vi "Code 0.0.2.vi"() -> ()   [LabVIEW 2017]
uses:
  <vilib>/Instr/_visa.llb/VISA Configure Serial Port (Instr).vi
panel:
  out "Error List":string
  in  "Flash Baudrate":u32(ring)=115200 items=["4800"=4800, "9600"=9600, "19200"=19200, "38400"=38400, "57600"=57600, "115200"=115200, "230400"=230400, "460800"=460800, "921600"=921600]
  in  "cmd Baudrate":u32(ring)=230400 items=["4800"=4800, "9600"=9600, "19200"=19200, "38400"=38400, "57600"=57600, "115200"=115200, "230400"=230400, "460800"=460800, "921600"=921600]
  in  "UUT COM Port":refnum<visa-resource-name>="COM4"
  in  "Next Button":bool
  in  "File Path Control":path
  out "Status":bool
  out "cmd Sent":bool
  out "CheckSumArray":u16[][](array[numeric]) format="%.0x"
  out "CheckSum":bool[][](array[boolean])
  in  "stop 9":bool
  in  "stop 8":bool
  out "CheckSum DataB":u16 format="%.0x"
  out "CheckSum Data":u16 format="%.0x"
  in  "stop 5":bool
  in  "stop 4":bool
  out "Array 3":u16[][](array[numeric]) format="%.0x"
  out "Num of Data packet":i32
  out "Writting Data":bool
  out "Size of Text File":i32
  out "Full Text File":u8[](array[numeric]) format="%.0x"
  out "All bytes in file in HEX U8":u8[](array[numeric]) format="%02x"
  out "Send Header":bool
  out "AutoBaud Success":bool
  out "sumHeader":u16 format="%.0x"
  in  "stop 3":bool
  in  "stop 2":bool
  out "error out":errorcluster
  in  "stop":bool
  out "Autobaud":string
  # "Ver 0.0.2"
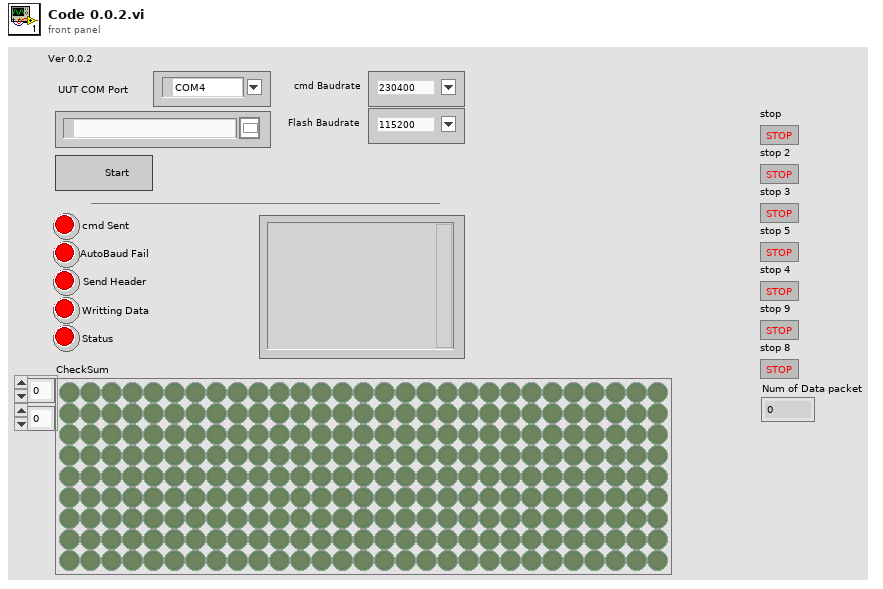
[diagram p1: front panel]
types:
  T1 = enum16{"open", "replace", "create", "open or create", "replace or create", "replace or create with confirmation"}
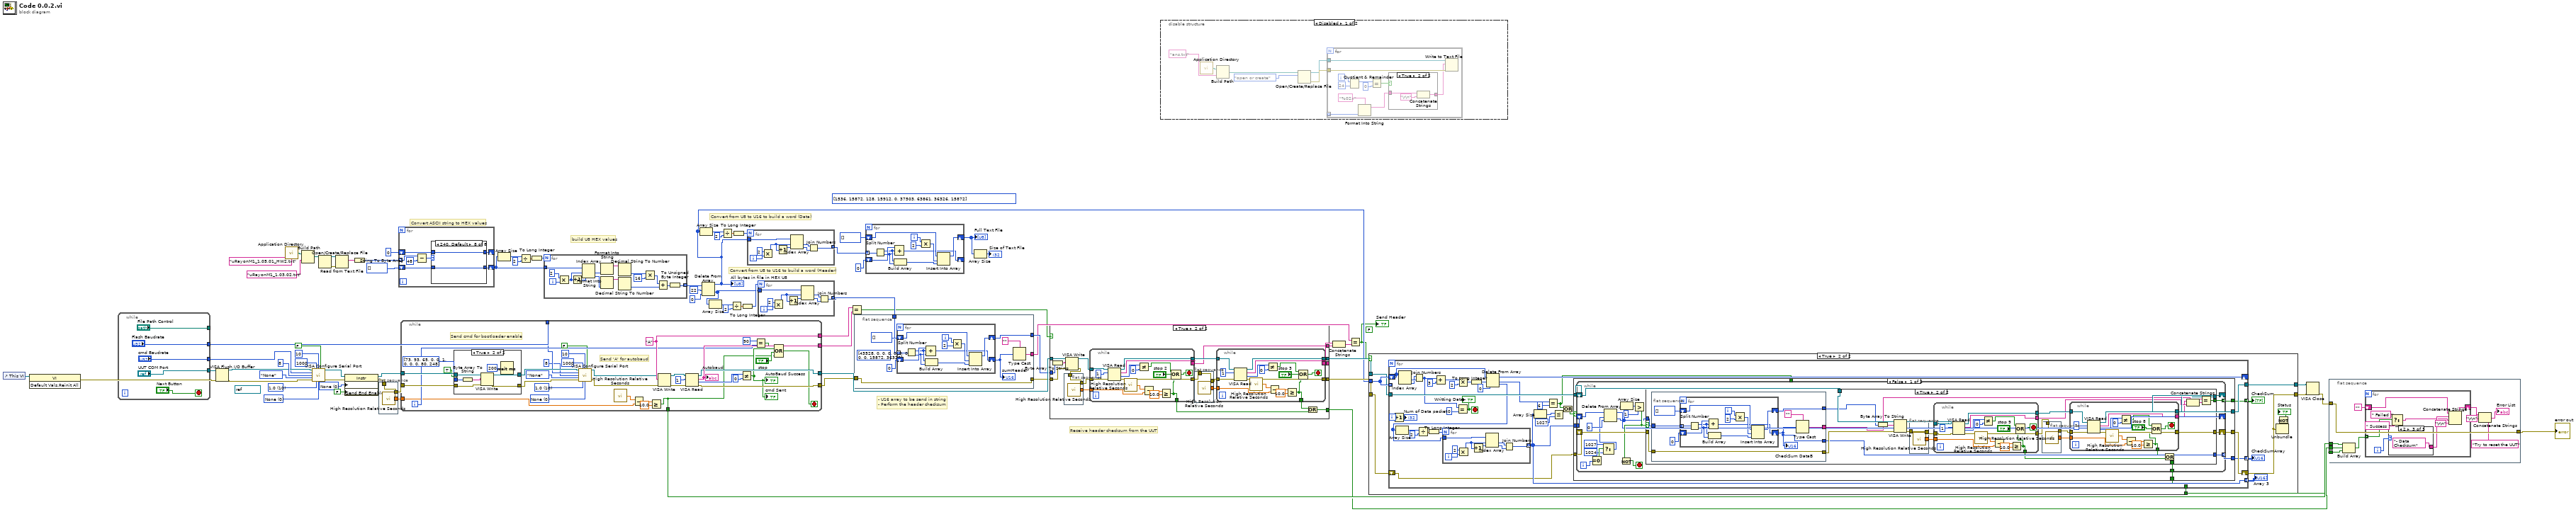
[diagram p0: block diagram]
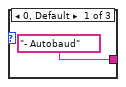
[diagram p2: hidden frame]
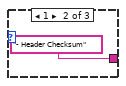
[diagram p3: hidden frame]
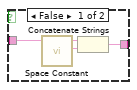
[diagram p5: hidden frame]
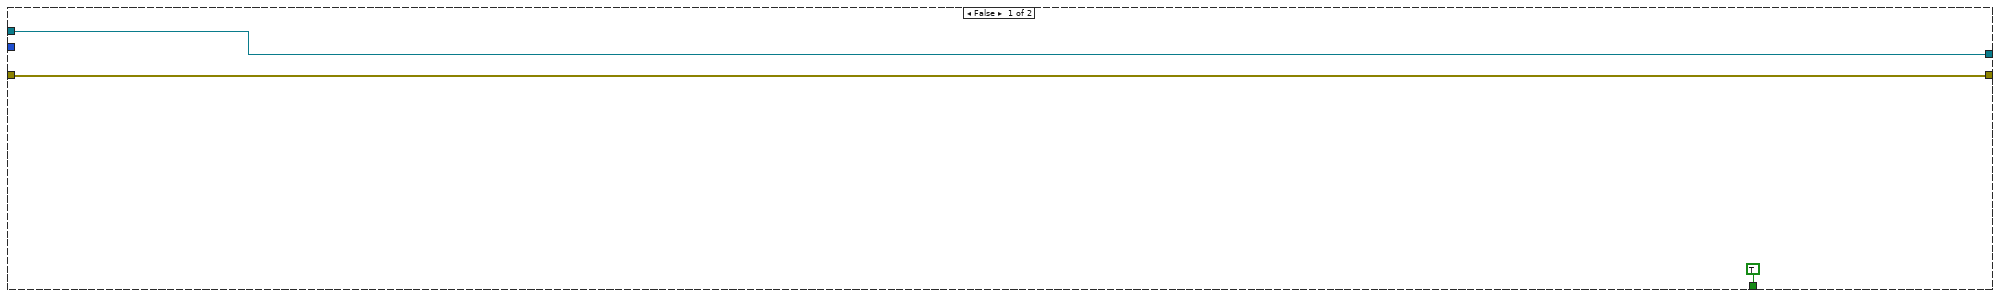
[diagram p7: hidden frame]
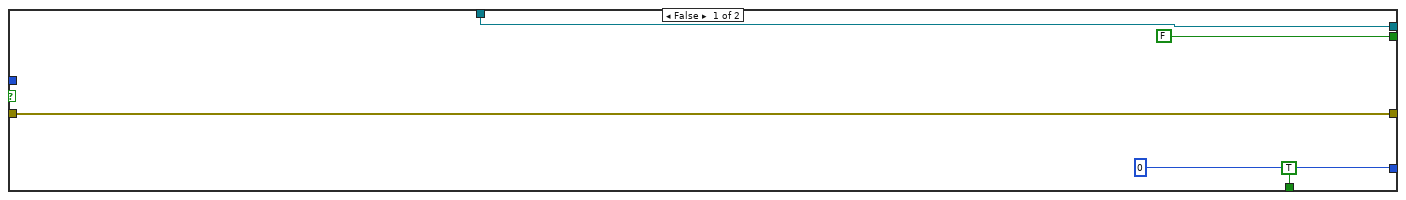
[diagram p8: hidden frame]
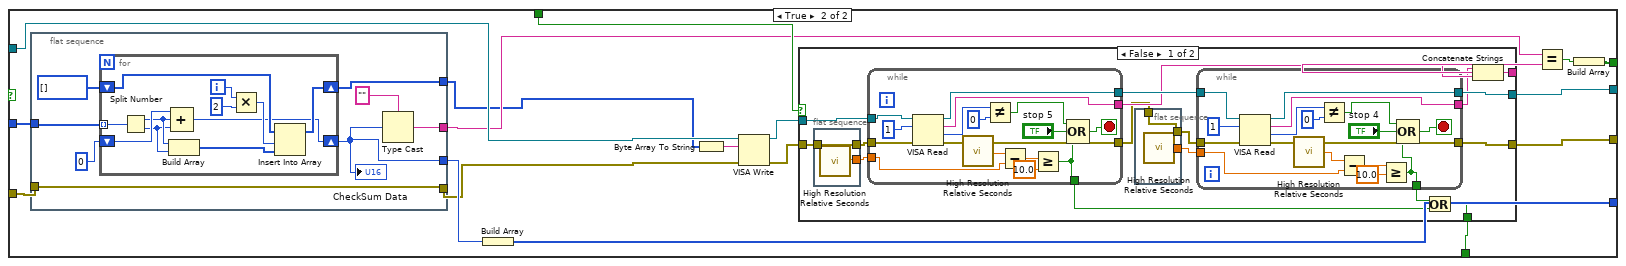
[diagram p9: hidden frame]
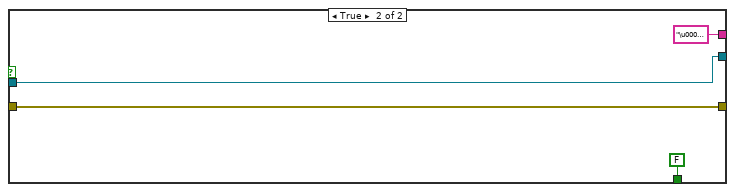
[diagram p10: hidden frame]
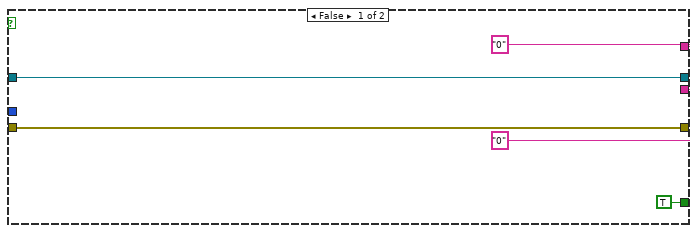
[diagram p11: hidden frame]
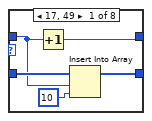
[diagram p12: hidden frame]
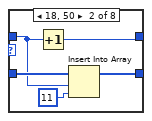
[diagram p13: hidden frame]
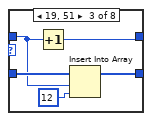
[diagram p14: hidden frame]
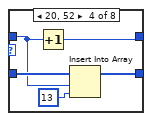
[diagram p15: hidden frame]
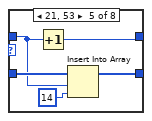
[diagram p16: hidden frame]
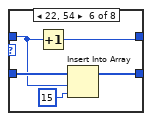
[diagram p17: hidden frame]
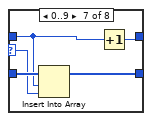
[diagram p18: hidden frame]
diagram:
  (unwired) FALSE
  (unwired) u16[] [1536, 15872, 128, 15912, 0, 37503, 63861, 36326, 15872] ("Array 4")
  (unwired) refnum<visa-resource-name> "COM4" ("VISA resource name")
  w39 = u16 0 items=["None", "LastBit", "TermChar", "Break"] ("Serial Settings:Serial End Mode for Writes")
  w43 = u16 0 items=["None", "XON/XOFF", "RTS/CTS", "XON/XOFF & RTS/CTS", "DTR/DSR", "XON/XOFF & DTR/DSR"] ("flow control (0:none)")
  w44 = u16 10 items=["1.0"=10, "1.5"=15, "2.0"=20] ("stop bits (10: 1 bit)")
  (unwired) "uRayonM1_1.05.01_HW2.txt" ("name or relative path")
  # "Receive header checksum from the UUT"
  # "- U16 array to be send in string\n- Perform the header checksum"
  # "Convert from U8 to U16 to build a word (Header)"
  # "build U8 HEX values"
  # "Convert from U8 to U16 to build a word (Data)"
  # "Convert ASCII string to HEX values"
  n1 = control-ref of="This VI"() -> (w15:refnum<vi>)
  n2 = invoke class="VI" method="Default Vals.Reinit All"(reference=w15) -> (error out=w18:errorcluster)  [unwired: 2 in, 2 out]
  n3 = while {
    tunnel: ["UUT COM Port"] -> w12
    tunnel: ["Flash Baudrate"] -> w11
    tunnel: ["cmd Baudrate"] -> w10
    tunnel: ["File Path Control"] -> _
    stop <- "Next Button" stop-if-true
  }
  n4 = VISA Flush I/O Buffer(VISA resource name=w12, error in (no error)=w18) -> (VISA resource name out=w16:refnum<visa-resource-name>, error out=w17:errorcluster)  [unwired: 1 in]
  n5 = call <vilib>:"Application Directory.vi"() -> ("Application Directory"=w70:path)
  n6 = Build Path(base path=w70, name or relative path="uRayonM1_1.03.02.txt") -> (appended path=w9:path)
  n7 = call-poly "VISA Configure Serial Port"("VISA resource name"=w16, "timeout (10sec)"=u32 1000, "termination char\n(0xA = '\\n' = LF)"=u8 10 ("termination char\n(0xA = '\\n' = LF)"), "Enable Termination\nChar (T)"=FALSE ("Enable Termination\nChar (T)"), "baud rate (9600)"=w10, "data bits (8)"=u16 8, "parity (0:none)"=enum16{"None", "Odd", "Even", "Mark", "Space"}."None", "error in (no error)"=w17, "stop bits (10: 1 bit)"=w44, "flow control (0:none)"=w43) -> ("VISA resource name out"=w41:refnum<visa-resource-name>, "error out"=w42:errorcluster)  [unwired: 4 in]
  n8 = Open/Create/Replace File(file path (use dialog)=w9) -> (refnum out=w68:refnum<file>, error out=w69:errorcluster)  [unwired: 5 in, 1 out]
  n9 = Read from Text File(file (use dialog)=w68, error in=w69) -> (text=w66:string)  [unwired: 2 in, 3 out]
  n10 = property class="Instr"(reference=w41, error in=w42, "Serial Settings:End Mode for Writes"=w39, "Message Based Settings:Send End Enable"=FALSE) -> (reference out=w14:refnum<visa-resource-name>, error out=w8:errorcluster)
  n11 = String To Byte Array(string=w66) -> (unsigned byte array=w67:u8[])
  n12 = flat-sequence {
    tunnel: w8 -> [w83]
    tunnel: [w83] -> w7
    tunnel: [w82] -> w6
    frame #0 {
      n13 = call <vilib>:"High Resolution Relative Seconds.vi"() -> ("relative seconds"=w82:dbl)
    }
  }
  n14 = for {
    tunnel: w67 -> [w90] mode=indexing
    shift-right: [w86] -> w63
    shift-left: u8[] [] -> [w87]
    shift-right: [w85] -> _
    shift-left: 0 ("y") -> [w84]
    n15 = Subtract(x=w90, y=u8 48) -> (x-y=w88:u8)
    n16 = case shown="240, Default" w88 {
      selector: w88 -> [_ _ _ _ _ _ w124 _]
      tunnel: [w93 w98 w104 w108 w113 w118 w123 w127] -> w86
      tunnel: w87 -> [w95 w99 w105 w110 w115 w120 w125 w127]
      tunnel: [w91 w96 w101 w106 w111 w116 w121 w126] -> w85
      tunnel: w84 -> [w92 w97 w102 w107 w112 w117 w122 w126]
      frame 17, 49 {
        n17 = Increment(x=w92) -> (x+1=w91:i32)
        n18 = Insert Into Array(array=w95, index=w92, new element=u8 10) -> (w93:u8[])
      }
      frame 18, 50 {
        n19 = Increment(x=w97) -> (x+1=w96:i32)
        n20 = Insert Into Array(array=w99, index=w97, new element=u8 11) -> (w98:u8[])
      }
      frame 19, 51 {
        n21 = Increment(x=w102) -> (x+1=w101:i32)
        n22 = Insert Into Array(array=w105, index=w102, new element=u8 12) -> (w104:u8[])
      }
      frame 20, 52 {
        n23 = Increment(x=w107) -> (x+1=w106:i32)
        n24 = Insert Into Array(array=w110, index=w107, new element=u8 13) -> (w108:u8[])
      }
      frame 21, 53 {
        n25 = Increment(x=w112) -> (x+1=w111:i32)
        n26 = Insert Into Array(array=w115, index=w112, new element=u8 14) -> (w113:u8[])
      }
      frame 22, 54 {
        n27 = Increment(x=w117) -> (x+1=w116:i32)
        n28 = Insert Into Array(array=w120, index=w117, new element=u8 15) -> (w118:u8[])
      }
      frame 0..9 {
        n29 = Insert Into Array(array=w125, index=w122, new element=w124) -> (w123:u8[])
        n30 = Increment(x=w122) -> (x+1=w121:i32)
      }
      frame 240, Default {
      }
    }
  }
  n31 = while {
    tunnel: [w163] -> w76
    tunnel: [w162] -> w75
    tunnel: w11 -> [w140]
    tunnel: w6 -> [w131]
    tunnel: w7 -> [w158]
    tunnel: [w160] -> w73
    tunnel: w14 -> [w159]
    tunnel: [w161] -> w74
    tunnel: [w128] -> w3
    i -> [w146]
    stop <- w149 stop-if-true
    w133 = u16 0 items=["None", "XON/XOFF", "RTS/CTS", "XON/XOFF & RTS/CTS", "DTR/DSR", "XON/XOFF & DTR/DSR"] ("flow control (0:none)")
    w134 = u16 10 items=["1.0"=10, "1.5"=15, "2.0"=20] ("stop bits (10: 1 bit)")
    w162 = "A" ("write buffer")
    # "Send cmd for bootloader enable"
    # "Send 'A' for autobaud"
    n32 = case shown="True" TRUE {
      tunnel: w159 -> [w165 w172]
      tunnel: w158 -> [w164 w171]
      tunnel: [w165 w170] -> w141
      tunnel: [w164 w169] -> w142
      tunnel: u8[] [73, 93, 65, 0, 0, 1, 0, 0, 0, 80, 248] ("output array") -> [_ w168]
      frame False {
      }
      frame True {
        n33 = Byte Array To String(unsigned byte array=w168) -> (string=w167:string)
        n34 = VISA Write(VISA resource name=w172, write buffer=w167, error in (no error)=w171) -> (VISA resource name out=w170:refnum<visa-resource-name>, error out=w169:errorcluster)  [unwired: 1 out]
        n35 = Wait (ms)(milliseconds to wait=u32 200) -> ()  [unwired: 1 out]
      }
    }
    n36 = call-poly "VISA Configure Serial Port"("VISA resource name"=w141, "timeout (10sec)"=u32 1000, "termination char\n(0xA = '\\n' = LF)"=u8 10 ("termination char\n(0xA = '\\n' = LF)"), "Enable Termination\nChar (T)"=FALSE ("Enable Termination\nChar (T)"), "baud rate (9600)"=w140, "data bits (8)"=u16 8, "parity (0:none)"=enum16{"None", "Odd", "Even", "Mark", "Space"}."None", "error in (no error)"=w142, "stop bits (10: 1 bit)"=w134, "flow control (0:none)"=w133) -> ("VISA resource name out"=w143:refnum<visa-resource-name>, "error out"=w144:errorcluster)  [unwired: 4 in]
    n37 = call <vilib>:"High Resolution Relative Seconds.vi"() -> ("relative seconds"=w132:dbl)
    n38 = Subtract(x=w132, y=w131) -> (x-y=w130:dbl)
    n39 = Greater Or Equal?(x=w130, y=10.0) -> (x >= y?=w128:bool)
    n40 = VISA Write(VISA resource name=w143, write buffer=w162, error in (no error)=w144) -> (VISA resource name out=w152:refnum<visa-resource-name>, error out=w151:errorcluster)  [unwired: 1 out]
    n41 = VISA Read(VISA resource name=w152, byte count=u32 1, error in (no error)=w151) -> (VISA resource name out=w161:refnum<visa-resource-name>, read buffer=w163:string, return count=w154:u32, error out=w160:errorcluster)
    "Autobaud" <- w163
    n42 = Not Equal?(x=w154, y=u32 0) -> (x != y?=w145:bool)
    "AutoBaud Success" <- w145
    "cmd Sent" <- w145
    n43 = Equal?(x=90, y=w146) -> (x = y?=w147:bool)
    n44 = Compound Arithmetic op=OR(w147, w145, "stop", w128) -> (w149:bool)
  }
  n45 = Array Size(array=w63) -> (size(s)=w62:i32)
  n46 = Divide(x=w62, y=2) -> (x/y=w60:dbl)
  n47 = To Long Integer(number=w60) -> (32bit integer=w59:i32)
  n48 = for {
    N: w59 -> [_]
    tunnel: w63 -> [w187]
    tunnel: [w173] -> w58 mode=indexing
    i -> [w186]
    n49 = Multiply(x=2, y=w186) -> (x*y=w184:i32)
    n50 = Increment(x=w184) -> (x+1=w183:i32)
    n51 = Index Array(array=w187, index #1=w184, index #2=w183) -> (element #1=w176:u8, element #2=w175:u8)
    n52 = Format Into String(w176) -> (resulting string=w177:string)  [unwired: 3 in, 1 out]
    n53 = Format Into String(w175) -> (resulting string=w182:string)  [unwired: 3 in, 1 out]
    n54 = Decimal String To Number(string=w177) -> (number=w178:i32)  [unwired: 2 in, 1 out]
    n55 = Decimal String To Number(string=w182) -> (number=w181:i32)  [unwired: 2 in, 1 out]
    n56 = Multiply(x=w178, y=16) -> (x*y=w180:i32)
    n57 = Add(x=w180, y=w181) -> (x+y=w174:i32)
    n58 = To Unsigned Byte Integer(number=w174) -> (unsigned 8bit integer=w173:u8)
  }
  n59 = Delete From Array(array=w58, length=22, index=0) -> (deleted portion=w29:u8[], array with subset deleted=w21:u8[])
  "All bytes in file in HEX U8" <- w21
  n60 = Array Size(array=w21) -> (size(s)=w35:i32)
  n61 = Array Size(array=w29) -> (size(s)=w34:i32)
  n62 = Divide(x=w35, y=2) -> (x/y=w37:dbl)
  n63 = Divide(x=w34, y=2) -> (x/y=w32:dbl)
  n64 = To Long Integer(number=w37) -> (32bit integer=w30:i32)
  n65 = To Long Integer(number=w32) -> (32bit integer=w31:i32)
  n66 = for {
    N: w30 -> [_]
    tunnel: w21 -> [w192]
    tunnel: [w188] -> w22 mode=indexing
    i -> [w191]
    n67 = Multiply(x=2, y=w191) -> (x*y=w194:i32)
    n68 = Increment(x=w194) -> (x+1=w195:i32)
    n69 = Index Array(array=w192, index #1=w194, index #2=w195) -> (element #1=w190:u8, element #2=w189:u8)
    n70 = Join Numbers(hi=w190, lo=w189) -> ((hi.lo)=w188:u16)
  }
  n71 = for {
    N: w31 -> [_]
    tunnel: w29 -> [w200]
    tunnel: [w196] -> w28 mode=indexing
    i -> [w199]
    n72 = Multiply(x=2, y=w199) -> (x*y=w202:i32)
    n73 = Increment(x=w202) -> (x+1=w203:i32)
    n74 = Index Array(array=w200, index #1=w202, index #2=w203) -> (element #1=w198:u8, element #2=w197:u8)
    n75 = Join Numbers(hi=w198, lo=w197) -> ((hi.lo)=w196:u16)
  }
  n76 = Equal?(x=w75, y=w76) -> (x = y?=w19:bool)
  n77 = flat-sequence {
    tunnel: w73 -> [w204]
    tunnel: [w209] -> w72
    tunnel: [w206] -> w71
    tunnel: w28 -> [w205]
    tunnel: [w204] -> w27
    frame #0 {
      (unwired) u16[] [43528, 0, 0, 0, 0, 0, 0, 0, 0, 15872, 36326]
      n78 = for {
        tunnel: w205 -> [w222] mode=indexing
        shift-right: [w217] -> w209
        shift-left: u8[] [] -> [w216]
        shift-right: [w214] -> w208
        shift-left: u16 0 -> [w215]
        i -> [w221]
        n79 = Split Number(x=w222) -> (hi(x)=w213:u8, lo(x)=w212:u8)
        n80 = Build Array(w213, w212) -> (w219:u8[])
        n81 = Compound Arithmetic op=ADD(w215, w213, w212) -> (w214:u16)
        n82 = Multiply(x=w221, y=2) -> (x*y=w218:i32)
        n83 = Insert Into Array(array=w216, index=w218, new element=w219) -> (w217:u8[])
      }
      "sumHeader" <- w208
      n84 = Type Cast(type="", x=w208) -> (*(type *) &x=w206:string)
    }
  }
  n85 = for {
    tunnel: w22 -> [w233] mode=indexing
    shift-right: [w228] -> w24
    shift-left: u8[] [] -> [w227]
    shift-right: [w225] -> _
    shift-left: u16 0 -> [w226]
    i -> [w232]
    n86 = Split Number(x=w233) -> (hi(x)=w224:u8, lo(x)=w223:u8)
    n87 = Build Array(w224, w223) -> (w230:u8[])
    n88 = Compound Arithmetic op=ADD(w226, w224, w223) -> (w225:u16)
    n89 = Multiply(x=w232, y=2) -> (x*y=w229:i32)
    n90 = Insert Into Array(array=w227, index=w229, new element=w230) -> (w228:u8[])
  }
  "Full Text File" <- w24
  n91 = Array Size(array=w24) -> (size(s)=→"Size of Text File":i32)
  n92 = case shown="True" w19 {
    tunnel: w27 -> [w237 w255]
    tunnel: w74 -> [w238 w254]
    tunnel: [w237 w253] -> w49
    tunnel: [w238 w252] -> w50
    tunnel: w72 -> [_ w251]
    tunnel: ["0" ("read buffer") w250] -> w53
    tunnel: ["0" ("read buffer") w249] -> w52
    tunnel: [TRUE w239] -> w2
    frame False {
    }
    frame True {
      n93 = Byte Array To String(unsigned byte array=w251) -> (string=w248:string)
      n94 = flat-sequence {
        tunnel: w247 -> [w261]
        tunnel: [w261] -> w246
        tunnel: [w260] -> w245
        frame #0 {
          n95 = call <vilib>:"High Resolution Relative Seconds.vi"() -> ("relative seconds"=w260:dbl)
        }
      }
      n96 = VISA Write(VISA resource name=w254, write buffer=w248, error in (no error)=w255) -> (VISA resource name out=w256:refnum<visa-resource-name>, error out=w247:errorcluster)  [unwired: 1 out]
      n97 = while {
        tunnel: w256 -> [w290]
        tunnel: [w291] -> w257
        tunnel: w246 -> [w289]
        tunnel: [w292] -> w244
        tunnel: [w283] -> w249
        tunnel: w245 -> [w279]
        tunnel: [w278] -> w240
        stop <- w285 stop-if-true
        n98 = VISA Read(VISA resource name=w290, byte count=u32 1, error in (no error)=w289) -> (VISA resource name out=w291:refnum<visa-resource-name>, read buffer=w283:string, return count=w284:u32, error out=w292:errorcluster)
        n99 = call <vilib>:"High Resolution Relative Seconds.vi"() -> ("relative seconds"=w280:dbl)
        n100 = Not Equal?(x=w284, y=u32 0) -> (x != y?=w287:bool)
        n101 = Subtract(x=w280, y=w279) -> (x-y=w281:dbl)
        n102 = Greater Or Equal?(x=w281, y=10.0) -> (x >= y?=w278:bool)
        n103 = Compound Arithmetic op=OR(w287, "stop 2", w278) -> (w285:bool)
      }
      n104 = flat-sequence {
        tunnel: w244 -> [w258]
        tunnel: [w258] -> _
        tunnel: [w259] -> w242
        tunnel: [w258] -> w243
        frame #0 {
          n105 = call <vilib>:"High Resolution Relative Seconds.vi"() -> ("relative seconds"=w259:dbl)
        }
      }
      n106 = while {
        tunnel: w257 -> [w276]
        tunnel: [w273] -> w252
        tunnel: w243 -> [w277]
        tunnel: [w274] -> w253
        tunnel: [w267] -> w250
        tunnel: w242 -> [w263]
        tunnel: [w262] -> w241
        stop <- w268 stop-if-true
        n107 = VISA Read(VISA resource name=w276, byte count=u32 1, error in (no error)=w277) -> (VISA resource name out=w273:refnum<visa-resource-name>, read buffer=w267:string, return count=w269:u32, error out=w274:errorcluster)
        n108 = call <vilib>:"High Resolution Relative Seconds.vi"() -> ("relative seconds"=w266:dbl)
        n109 = Not Equal?(x=w269, y=u32 0) -> (x != y?=w272:bool)
        n110 = Subtract(x=w266, y=w263) -> (x-y=w265:dbl)
        n111 = Greater Or Equal?(x=w265, y=10.0) -> (x >= y?=w262:bool)
        n112 = Compound Arithmetic op=OR(w272, "stop 3", w262) -> (w268:bool)
      }
      n113 = Or(x=w241, y=w240) -> (x .or. y?=w239:bool)
    }
  }
  n114 = disable-structure shown="Disabled" {
    frame Disabled {
      n115 = call <vilib>:"Application Directory.vi"() -> ("Application Directory"=w298:path)
      n116 = Build Path(base path=w298, name or relative path="ans.txt") -> (appended path=w297:path)
      n117 = Open/Create/Replace File(file path (use dialog)=w297, operation (0:open)=T1."open or create") -> (refnum out=w294:refnum<file>, error out=w295:errorcluster)  [unwired: 4 in, 1 out]
      n118 = for {
        tunnel: _ -> [w310] mode=indexing
        tunnel: w295 -> [w308]
        tunnel: w294 -> [w307]
        i -> [w303]
        n119 = Quotient & Remainder(x=w303, y=24 ("x")) -> (x-y*floor(x/y)=w301:i32)  [unwired: 1 out]
        n120 = Format Into String(format string="%02x", w310) -> (resulting string=w306:string)  [unwired: 2 in, 1 out]
        n121 = Equal?(x=w301, y=0) -> (x = y?=w304:bool)
        n122 = case shown="True" w304 {
          tunnel: w306 -> [w313 w316]
          tunnel: [w312 w315] -> w305
          frame False {
            n123 = call <vilib>:"Space Constant.vi"() -> ("String"=w311:string)
            n124 = Concatenate Strings(w313, w311) -> (w312:string)
          }
          frame True {
            n125 = Concatenate Strings(w316, "\r\n") -> (w315:string)
          }
        }
        n126 = Write to Text File(file (use dialog)=w307, text=w305, error in=w308) -> ()  [unwired: 1 in, 3 out]
      }
    }
    frame Enabled {
    }
  }
  n127 = Concatenate Strings(w53, w52) -> (w51:string)
  n128 = Equal?(x=w71, y=w51) -> (x = y?=w20:bool)
  "Send Header" <- w20
  n129 = case shown="True" w20 {
    tunnel: w50 -> [w319 w328]
    tunnel: w49 -> [w318 w324]
    tunnel: [w319 w327] -> w55
    tunnel: [w318 w323] -> w54
    tunnel: w21 -> [_ w329]
    tunnel: [TRUE w320] -> w1
    frame False {
    }
    frame True {
      n130 = for {
        shift-right: [w353] -> _
        shift-left: w329 -> [w364]
        tunnel: w329 -> [_] mode=indexing
        tunnel: [w346] -> w330 mode=indexing
        tunnel: w328 -> [w345]
        tunnel: [w341] -> w327
        tunnel: [w339] -> w326 mode=indexing
        tunnel: [w338] -> w325 mode=indexing
        shift-right: [w340] -> w323
        shift-left: w324 -> [w332]
        tunnel: [w331] -> w320
        i -> [w354]
        stop <- w357 stop-if-true
        n131 = Increment(x=w354) -> (x+1=→"Num of Data packet":i32)
        n132 = Index Array(array=w364) -> (element #1=w363:u8, element #2=w362:u8)  [unwired: 2 in]
        n133 = Join Numbers(hi=w362, lo=w363) -> ((hi.lo)=w334:u16)
        n134 = Add(x=w334, y=u32 3) -> (x+y=w360:u32)
        n135 = Equal?(x=w334, y=u16 0) -> (x = y?=w357:bool)
        "Writting Data" <- w357
        n136 = Multiply(x=w360, y=u32 2) -> (x*y=w358:u32)
        n137 = To Long Integer(number=w358) -> (32bit integer=w335:i32)
        n138 = Delete From Array(array=w364, length=w335, index=0) -> (deleted portion=w336:u8[], array with subset deleted=w353:u8[])
        n139 = Array Size(array=w336) -> (size(s)=w350:i32)
        n140 = Divide(x=w350, y=2) -> (x/y=w352:dbl)
        n141 = To Long Integer(number=w352) -> (32bit integer=w349:i32)
        n142 = for {
          N: w349 -> [_]
          tunnel: w336 -> [w575]
          tunnel: [w571] -> w346 mode=indexing
          i -> [w574]
          n143 = Multiply(x=2, y=w574) -> (x*y=w577:i32)
          n144 = Increment(x=w577) -> (x+1=w578:i32)
          n145 = Index Array(array=w575, index #1=w577, index #2=w578) -> (element #1=w573:u8, element #2=w572:u8)
          n146 = Join Numbers(hi=w573, lo=w572) -> ((hi.lo)=w571:u16)
        }
        n147 = Array Size(array=w346) -> (size(s)=w348:i32)
        n148 = Equal?(x=w335, y=6) -> (x = y?=w333:bool)
        n149 = Less Or Equal?(x=w348, y=1027) -> (x <= y?=w343:bool)
        n150 = Or(x=w333, y=w343) -> (x .or. y?=w342:bool)
        n151 = case shown="False" w342 {
          tunnel: w332 -> [w369 w492]
          tunnel: w345 -> [w372 w483]
          tunnel: [w371 w495] -> w340
          tunnel: [w370 w494] -> w341
          tunnel: w346 -> [w367 w493]
          tunnel: [w368 w489] -> w339
          tunnel: [w366 w487] -> w338
          tunnel: w333 -> [_ w486]
          tunnel: [w365 w478] -> w331
          frame False {
            n152 = while {
              tunnel: w367 -> [_]
              tunnel: [w388] -> w368 mode=indexing
              shift-right: [w390] -> w370
              shift-left: w372 -> [w392]
              shift-right: [w391] -> w371
              shift-left: w369 -> [w389]
              shift-right: [w380] -> _
              shift-left: w367 -> [w387]
              tunnel: [w379] -> w366 mode=indexing
              tunnel: [w373] -> w365
              i -> [w378]
              stop <- w382 stop-if-true
              n153 = Equal To 0?(x=w378) -> (x = 0?=w377:bool)
              n154 = Select(t=1027 ("length"), s=w377, f=1024 ("length")) -> (s? t:f=w374:i32)
              n155 = Delete From Array(array=w387, length=w374, index=0) -> (deleted portion=w381:u16[], array with subset deleted=w380:u16[])
              n156 = Array Size(array=w381) -> (size(s)=w385:i32)
              n157 = Greater?(x=w385, y=1) -> (0:w383:bool)
              n158 = Not(x=w383) -> (.not. x?=w382:bool)
              n159 = case shown="True" w383 {
                tunnel: w392 -> [w395 w421]
                tunnel: [w397 w420] -> w391
                tunnel: [w395 w419] -> w390
                tunnel: w389 -> [w397 w417]
                tunnel: [FALSE w412] -> w388
                tunnel: w381 -> [_ w411]
                tunnel: [u16 0 ("Numeric") w410] -> w379
                tunnel: [TRUE w398] -> w373
                frame False {
                }
                frame True {
                  n160 = flat-sequence {
                    tunnel: w417 -> [w428]
                    tunnel: [w432] -> w408
                    tunnel: [w430] -> w413
                    tunnel: w411 -> [w429]
                    tunnel: [w428] -> w418
                    tunnel: [w427] -> w410
                    frame #0 {
                      n161 = for {
                        tunnel: w429 -> [w445] mode=indexing
                        shift-right: [w440] -> w432
                        shift-left: u8[] [] -> [w439]
                        shift-right: [w437] -> w427
                        shift-left: u16 0 -> [w438]
                        i -> [w444]
                        n162 = Split Number(x=w445) -> (hi(x)=w436:u8, lo(x)=w435:u8)
                        n163 = Build Array(w436, w435) -> (w442:u8[])
                        n164 = Compound Arithmetic op=ADD(w438, w436, w435) -> (w437:u16)
                        n165 = Multiply(x=w444, y=2) -> (x*y=w441:i32)
                        n166 = Insert Into Array(array=w439, index=w441, new element=w442) -> (w440:u8[])
                      }
                      "CheckSum DataB" <- w427
                      n167 = Type Cast(type="", x=w427) -> (*(type *) &x=w430:string)
                    }
                  }
                  n168 = Byte Array To String(unsigned byte array=w408) -> (string=w409:string)
                  n169 = VISA Write(VISA resource name=w421, write buffer=w409, error in (no error)=w418) -> (VISA resource name out=w404:refnum<visa-resource-name>, error out=w403:errorcluster)  [unwired: 1 out]
                  n170 = flat-sequence {
                    tunnel: [w426] -> w401
                    tunnel: w403 -> [w425]
                    tunnel: [w425] -> w402
                    frame #0 {
                      n171 = call <vilib>:"High Resolution Relative Seconds.vi"() -> ("relative seconds"=w426:dbl)
                    }
                  }
                  n172 = while {
                    tunnel: w404 -> [w474]
                    tunnel: [w475] -> w422
                    tunnel: [w476] -> w405
                    tunnel: [w468] -> w416
                    tunnel: w402 -> [w464]
                    tunnel: w401 -> [w463]
                    tunnel: [w462] -> w399
                    stop <- w470 stop-if-true
                    n173 = VISA Read(VISA resource name=w474, byte count=u32 1, error in (no error)=w464) -> (VISA resource name out=w475:refnum<visa-resource-name>, read buffer=w468:string, return count=w469:u32, error out=w476:errorcluster)
                    n174 = call <vilib>:"High Resolution Relative Seconds.vi"() -> ("relative seconds"=w465:dbl)
                    n175 = Not Equal?(x=w469, y=u32 0) -> (x != y?=w472:bool)
                    n176 = Subtract(x=w465, y=w463) -> (x-y=w466:dbl)
                    n177 = Greater Or Equal?(x=w466, y=10.0) -> (x >= y?=w462:bool)
                    n178 = Compound Arithmetic op=OR(w472, "stop 9", w462) -> (w470:bool)
                  }
                  n179 = flat-sequence {
                    tunnel: w405 -> [w424]
                    tunnel: [w424] -> w406
                    tunnel: [w423] -> w407
                    frame #0 {
                      n180 = call <vilib>:"High Resolution Relative Seconds.vi"() -> ("relative seconds"=w423:dbl)
                    }
                  }
                  n181 = while {
                    tunnel: w422 -> [w460]
                    tunnel: [w457] -> w419
                    tunnel: w406 -> [w461]
                    tunnel: [w458] -> w420
                    tunnel: [w451] -> w415
                    tunnel: w407 -> [w447]
                    tunnel: [w446] -> w400
                    stop <- w452 stop-if-true
                    n182 = VISA Read(VISA resource name=w460, byte count=u32 1, error in (no error)=w461) -> (VISA resource name out=w457:refnum<visa-resource-name>, read buffer=w451:string, return count=w453:u32, error out=w458:errorcluster)
                    n183 = call <vilib>:"High Resolution Relative Seconds.vi"() -> ("relative seconds"=w450:dbl)
                    n184 = Not Equal?(x=w453, y=u32 0) -> (x != y?=w456:bool)
                    n185 = Subtract(x=w450, y=w447) -> (x-y=w449:dbl)
                    n186 = Greater Or Equal?(x=w449, y=10.0) -> (x >= y?=w446:bool)
                    n187 = Compound Arithmetic op=OR(w456, "stop 8", w446) -> (w452:bool)
                  }
                  n188 = Or(x=w400, y=w399) -> (x .or. y?=w398:bool)
                  n189 = Concatenate Strings(w415, w416) -> (w414:string)
                  n190 = Equal?(x=w413, y=w414) -> (x = y?=w412:bool)
                }
              }
            }
          }
          frame True {
            n191 = flat-sequence {
              tunnel: w492 -> [w553]
              tunnel: [w557] -> w479
              tunnel: [w555] -> w481
              tunnel: w493 -> [w554]
              tunnel: [w553] -> w482
              tunnel: [w552] -> w488
              frame #0 {
                n192 = for {
                  tunnel: w554 -> [w570] mode=indexing
                  shift-right: [w565] -> w557
                  shift-left: u8[] [] -> [w564]
                  shift-right: [w562] -> w552
                  shift-left: u16 0 -> [w563]
                  i -> [w569]
                  n193 = Split Number(x=w570) -> (hi(x)=w561:u8, lo(x)=w560:u8)
                  n194 = Build Array(w561, w560) -> (w567:u8[])
                  n195 = Compound Arithmetic op=ADD(w563, w561, w560) -> (w562:u16)
                  n196 = Multiply(x=w569, y=2) -> (x*y=w566:i32)
                  n197 = Insert Into Array(array=w564, index=w566, new element=w567) -> (w565:u8[])
                }
                "CheckSum Data" <- w552
                n198 = Type Cast(type="", x=w552) -> (*(type *) &x=w555:string)
              }
            }
            n199 = Build Array(w488) -> (w487:u16[])
            n200 = Byte Array To String(unsigned byte array=w479) -> (string=w480:string)
            n201 = VISA Write(VISA resource name=w483, write buffer=w480, error in (no error)=w482) -> (VISA resource name out=w484:refnum<visa-resource-name>, error out=w485:errorcluster)  [unwired: 1 out]
            n202 = case shown="False" w486 {
              tunnel: w484 -> [w510 w550]
              tunnel: w485 -> [w503 w549]
              tunnel: [w509 w549] -> w495
              tunnel: [w508 w550] -> w494
              tunnel: [w505 "\u0000\u0000"] -> w491
              tunnel: [w496 FALSE] -> w478
              frame False {
                n203 = flat-sequence {
                  tunnel: [w515] -> w504
                  tunnel: w503 -> [w514]
                  tunnel: [w514] -> w502
                  frame #0 {
                    n204 = call <vilib>:"High Resolution Relative Seconds.vi"() -> ("relative seconds"=w515:dbl)
                  }
                }
                n205 = while {
                  tunnel: w510 -> [w544]
                  tunnel: [w545] -> w511
                  tunnel: w502 -> [w543]
                  tunnel: [w546] -> w501
                  tunnel: [w537] -> w507
                  tunnel: w504 -> [w535]
                  tunnel: [w532] -> w497
                  stop <- w539 stop-if-true
                  n206 = VISA Read(VISA resource name=w544, byte count=u32 1, error in (no error)=w543) -> (VISA resource name out=w545:refnum<visa-resource-name>, read buffer=w537:string, return count=w538:u32, error out=w546:errorcluster)
                  n207 = call <vilib>:"High Resolution Relative Seconds.vi"() -> ("relative seconds"=w536:dbl)
                  n208 = Not Equal?(x=w538, y=u32 0) -> (x != y?=w541:bool)
                  n209 = Subtract(x=w536, y=w535) -> (x-y=w534:dbl)
                  n210 = Greater Or Equal?(x=w534, y=10.0) -> (x >= y?=w532:bool)
                  n211 = Compound Arithmetic op=OR(w541, "stop 5", w532) -> (w539:bool)
                }
                n212 = flat-sequence {
                  tunnel: w501 -> [w513]
                  tunnel: [w513] -> w500
                  tunnel: [w512] -> w499
                  frame #0 {
                    n213 = call <vilib>:"High Resolution Relative Seconds.vi"() -> ("relative seconds"=w512:dbl)
                  }
                }
                n214 = while {
                  tunnel: w511 -> [w530]
                  tunnel: [w527] -> w508
                  tunnel: w500 -> [w531]
                  tunnel: [w528] -> w509
                  tunnel: [w521] -> w506
                  tunnel: w499 -> [w517]
                  tunnel: [w516] -> w498
                  stop <- w522 stop-if-true
                  n215 = VISA Read(VISA resource name=w530, byte count=u32 1, error in (no error)=w531) -> (VISA resource name out=w527:refnum<visa-resource-name>, read buffer=w521:string, return count=w523:u32, error out=w528:errorcluster)
                  n216 = call <vilib>:"High Resolution Relative Seconds.vi"() -> ("relative seconds"=w518:dbl)
                  n217 = Not Equal?(x=w523, y=u32 0) -> (x != y?=w526:bool)
                  n218 = Subtract(x=w518, y=w517) -> (x-y=w519:dbl)
                  n219 = Greater Or Equal?(x=w519, y=10.0) -> (x >= y?=w516:bool)
                  n220 = Compound Arithmetic op=OR(w526, "stop 4", w516) -> (w522:bool)
                }
                n221 = Or(x=w498, y=w497) -> (x .or. y?=w496:bool)
                n222 = Concatenate Strings(w506, w507) -> (w505:string)
              }
              frame True {
              }
            }
            n223 = Equal?(x=w481, y=w491) -> (x = y?=w490:bool)
            n224 = Build Array(w490) -> (w489:bool[])
          }
        }
      }
      "Array 3" <- w330
      "CheckSum" <- w326
      "CheckSumArray" <- w325
      n225 = Unbundle(w323) -> ("status"=w322:bool)  [unwired: 2 out]
      n226 = Not(x=w322) -> (.not. x?=→"Status":bool)
    }
  }
  n227 = VISA Close(VISA resource name=w55, error in (no error)=w54) -> (error out=w5:errorcluster)
  n228 = flat-sequence {
    tunnel: w5 -> [w588]
    tunnel: [w588] -> w4
    tunnel: w3 -> [w587]
    tunnel: w2 -> [w586]
    tunnel: w1 -> [w585]
    frame #0 {
      n229 = Build Array(w587, w586, w585) -> (w584:bool[])
      n230 = for {
        tunnel: w584 -> [w597] mode=indexing
        shift-right: [w595] -> w582
        shift-left: "" -> [w596]
        i -> [w593]
        n231 = case shown="2" w593 {
          tunnel: ["- Autobaud" "- Header Checksum" "- Data Checksum"] -> w590
          frame 0, Default {
          }
          frame 1 {
          }
          frame 2 {
          }
        }
        n232 = Select(t=" Failed !", s=w597, f=" Success !") -> (s? t:f=w589:string)
        n233 = Concatenate Strings(w596, w590, w589, "\r\n") -> (w595:string)
      }
      n234 = Concatenate Strings(w582, "\r\n", "Try to reset the UUT" ("string")) -> (→"Error List":string)
    }
  }
  "error out" <- w4
